vi "Create Command.vi"(10 "Command Queue":refnum<queue>) -> (3 "Stop.lvclass":refnum<class "Stop.lvclass">)   [LabVIEW 2010, in "Stop.lvclass"]
doc: "This instance of Create Command.vi writes the value of the Command Queue reference to the data stored within Stop.lvclass."
uses:
  Stop.lvclass
  Application Command/Application Command.lvclass
  Stop.lvclass/Stop.ctl
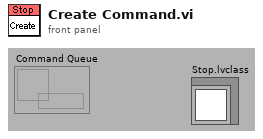
[diagram p1: front panel]
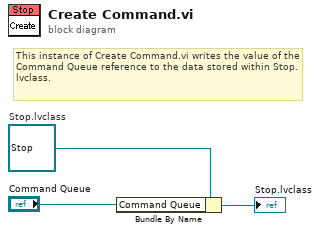
[diagram p0: block diagram]
diagram:
  w3 = refnum<class "Stop.lvclass"> refnum  # Stop.lvclass
  # "This instance of Create Command.vi writes the value of the  Command Queue reference to the data stored within Stop.lvclass."
  n1 = Bundle By Name "Bundle By Name"(cluster=w3, "Command Queue"="Command Queue") -> (→"Stop.lvclass":refnum<class "Stop.lvclass">)
